vi "Create Child Nodes.vi"(1 "Pmin (parent)":sgl[](array[numeric]), 2 "Pmax (parent)":sgl[](array[numeric]), 3 "Parent":i32=-1, 4 "Level (parent+1)":i32=-1) -> (0 "8 Child nodes array":T1[](array[typedef]))   [LabVIEW 2014]
uses:
  Typedefs/TreeNodeBox.ctl
  Typedefs/Quad.ctl
panel:
  # "PN 17/01/2015"
  # "Vertices"
  # "Edges"
  # "Unit normal"
  # "Edge unit normals"
  # "Vertices"
  # "Edges"
  # "Unit normal"
  # "Edge unit normals"
  # "Vertices"
  # "Edges"
  # "Unit normal"
  # "Edge unit normals"
  # "Vertices"
  # "Edges"
  # "Unit normal"
  # "Edge unit normals"
  # "Vertices"
  # "Edges"
  # "Unit normal"
  # "Edge unit normals"
  # "Vertices"
  # "Edges"
  # "Unit normal"
  # "Edge unit normals"
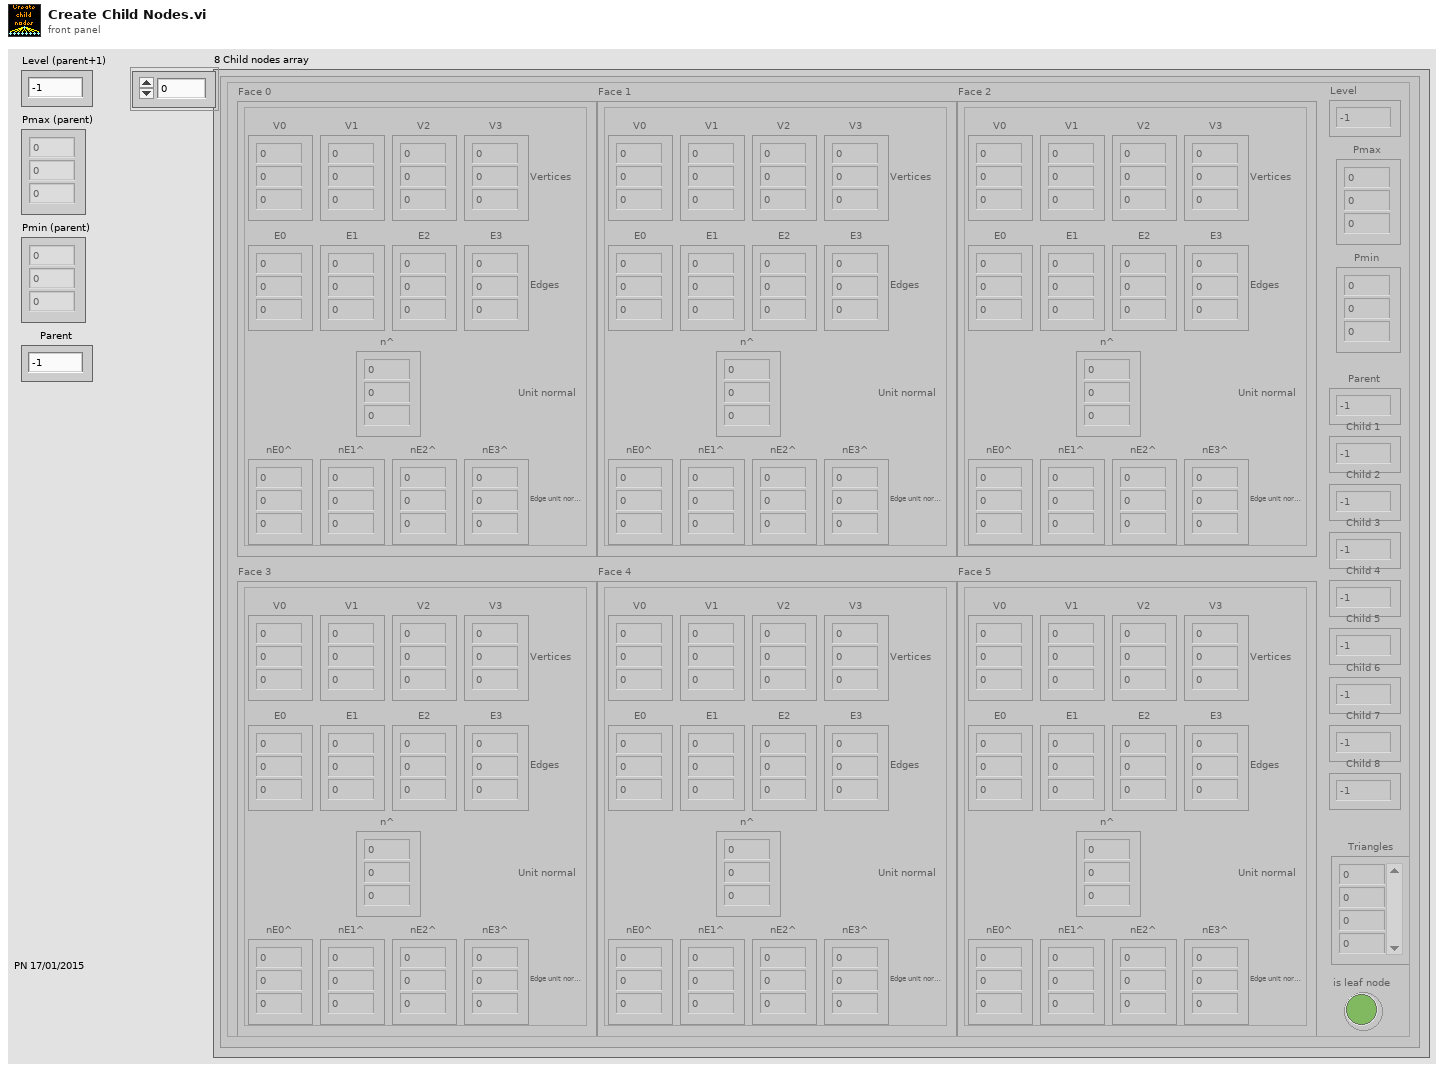
[diagram p1: front panel]
types:
  T1 = typedef "TreeNodeBox.ctl" = cluster{"Face 0":T2, "Face 1":T2, "Face 2":T2, "Face 3":T2, "Face 4":T2, "Face 5":T2, "Level":i32, "Pmax":sgl[], "Pmin":sgl[], "Parent":i32, "Child 1":i32, "Child 2":i32, "Child 3":i32, "Child 4":i32, "Child 5":i32, "Child 6":i32, "Child 7":i32, "Child 8":i32, "Triangles":i32[], "is leaf node":bool}
  T2 = typedef "Quad.ctl" = cluster{"V0":sgl[], "V1":sgl[], "V2":sgl[], "V3":sgl[], "E0":sgl[], "E1":sgl[], "E2":sgl[], "E3":sgl[], "n^":sgl[], "nE0^":sgl[], "nE1^":sgl[], "nE2^":sgl[], "nE3^":sgl[]}
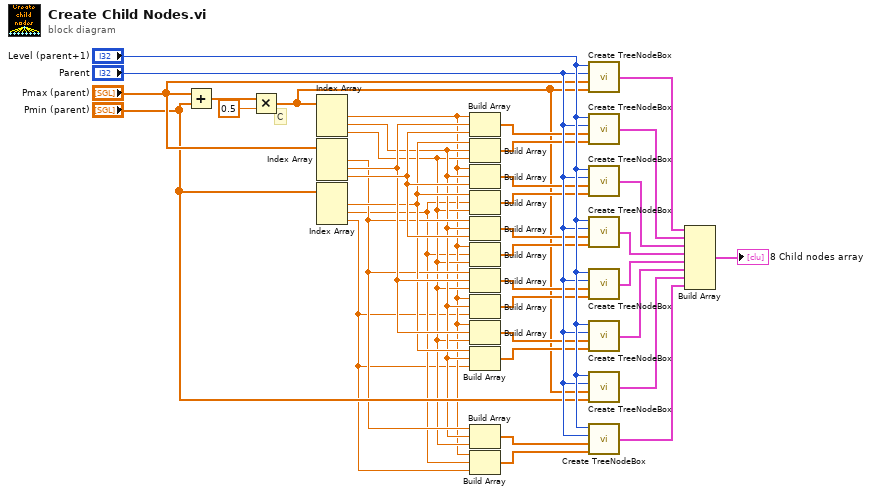
[diagram p0: block diagram]
diagram:
  # "C"
  n1 = Add(x="Pmax (parent)", y="Pmin (parent)") -> (x+y=w36:sgl[])
  n2 = Multiply(x=w36, y=sgl 0.5) -> (x*y=w19:sgl[])
  n3 = Index Array(array=w19) -> (element #1=w12:sgl, element #2=w14:sgl, element #3=w13:sgl)  [unwired: 3 in]
  n4 = Index Array(array="Pmax (parent)") -> (element #1=w15:sgl, element #2=w23:sgl, element #3=w26:sgl)  [unwired: 3 in]
  n5 = Index Array(array="Pmin (parent)") -> (element #1=w21:sgl, element #2=w11:sgl, element #3=w10:sgl)  [unwired: 3 in]
  n6 = Build Array(w12, w23, w26) -> (w32:sgl[])
  n7 = Build Array(w21, w14, w13) -> (w31:sgl[])
  n8 = Build Array(w12, w14, w26) -> (w30:sgl[])
  n9 = Build Array(w21, w11, w13) -> (w29:sgl[])
  n10 = Build Array(w15, w14, w26) -> (w28:sgl[])
  n11 = Build Array(w12, w11, w13) -> (w27:sgl[])
  n12 = Build Array(w15, w23, w13) -> (w25:sgl[])
  n13 = Build Array(w12, w14, w10) -> (w24:sgl[])
  n14 = Build Array(w12, w23, w13) -> (w22:sgl[])
  n15 = Build Array(w21, w14, w10) -> (w20:sgl[])
  n16 = Build Array(w15, w14, w13) -> (w17:sgl[])
  n17 = Build Array(w12, w11, w10) -> (w16:sgl[])
  n18 = call "Create TreeNodeBox.vi"("Pmin"=w19, "Pmax"="Pmax (parent)", "Parent"="Parent", "Level"="Level (parent+1)") -> ("Box"=w9:T1)
  n19 = call "Create TreeNodeBox.vi"("Pmin"=w31, "Pmax"=w32, "Parent"="Parent", "Level"="Level (parent+1)") -> ("Box"=w8:T1)
  n20 = call "Create TreeNodeBox.vi"("Pmin"=w29, "Pmax"=w30, "Parent"="Parent", "Level"="Level (parent+1)") -> ("Box"=w7:T1)
  n21 = call "Create TreeNodeBox.vi"("Pmin"=w27, "Pmax"=w28, "Parent"="Parent", "Level"="Level (parent+1)") -> ("Box"=w6:T1)
  n22 = call "Create TreeNodeBox.vi"("Pmin"=w24, "Pmax"=w25, "Parent"="Parent", "Level"="Level (parent+1)") -> ("Box"=w5:T1)
  n23 = call "Create TreeNodeBox.vi"("Pmin"=w20, "Pmax"=w22, "Parent"="Parent", "Level"="Level (parent+1)") -> ("Box"=w4:T1)
  n24 = call "Create TreeNodeBox.vi"("Pmin"="Pmin (parent)", "Pmax"=w19, "Parent"="Parent", "Level"="Level (parent+1)") -> ("Box"=w3:T1)
  n25 = call "Create TreeNodeBox.vi"("Pmin"=w16, "Pmax"=w17, "Parent"="Parent", "Level"="Level (parent+1)") -> ("Box"=w2:T1)
  n26 = Build Array(w9, w8, w7, w6, w5, w4, w3, w2) -> (→"8 Child nodes array":T1[])
